vi "Request Data JSON.vi"(8 "error in (no error)":errorcluster, 11 "GetInputDefaultSettings in":refnum<class "GetInputDefaultSettings.lvclass">) -> (0 "error out":errorcluster, 2 "Request Data JSON":string, 3 "GetInputDefaultSettings out":refnum<class "GetInputDefaultSettings.lvclass">)   [LabVIEW 2020, in "obs-websocket.lvlib" / "GetInputDefaultSettings.lvclass"]
uses:
  GetInputDefaultSettings.lvclass
  GetInputDefaultSettings.lvclass/GetInputDefaultSettings.ctl
  96b8c802-6b60-4e66-bebe-91fdfc631dc3.vi
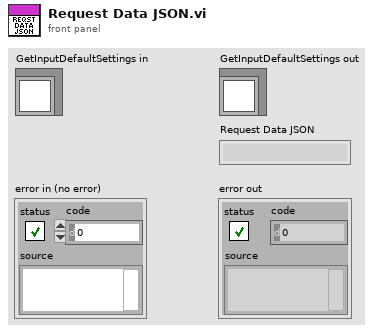
[diagram p1: front panel]
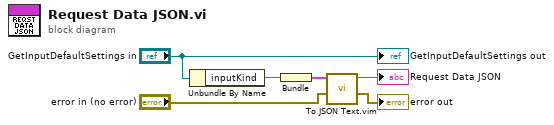
[diagram p0: block diagram]
diagram:
  n1 = Unbundle By Name("GetInputDefaultSettings in") -> ("inputKind"=w5:string)
  n2 = Bundle("inputKind"=w5) -> (w4:cluster{"inputKind":string})  [unwired: 1 in]
  n3 = call "To JSON Text.vim"("error in (no error)"="error in (no error)", "Anything"=w4) -> ("error out"=→"error out":errorcluster, "<JSON>"=→"Request Data JSON":string)  [unwired: 8 in]
  "GetInputDefaultSettings out" <- "GetInputDefaultSettings in"
